vi "Initialize.vi"(8 "error in (no error)":errorcluster caption="错误输入（无错误）", 11 "VISA resource name in":refnum<visa-resource-name> caption="VISA资源名称输入") -> (0 "error out":errorcluster caption="错误输出", 3 "VISA resource name out":refnum<visa-resource-name> caption="VISA资源名称输出")   [LabVIEW 2015]
uses:
  <vilib>/Instr/_visa.llb/VISA Configure Serial Port (Instr).vi
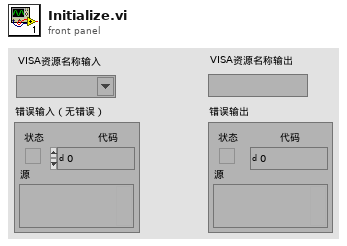
[diagram p1: front panel]
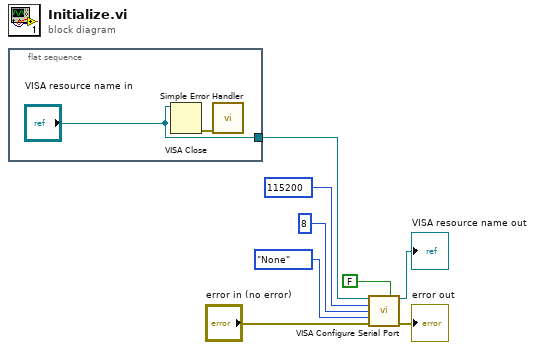
[diagram p0: block diagram]
diagram:
  n1 = flat-sequence {
    tunnel: ["VISA resource name in"] -> w4
    frame #0 {
      n2 = VISA Close(VISA resource name="VISA resource name in") -> (error out=w10:errorcluster)  [unwired: 1 in]
      n3 = call <vilib>:"Simple Error Handler.vi"("error in (no error)"=w10) -> ()  [unwired: 4 in, 5 out]
    }
  }
  n4 = call-poly "VISA Configure Serial Port"("VISA resource name"=w4, "Enable Termination\nChar (T)"=FALSE ("Enable Termination\nChar (T)"), "baud rate (9600)"=u32 115200, "data bits (8)"=u16 8, "parity (0:none)"=enum16{"None", "Odd", "Even", "Mark", "Space"}."None", "error in (no error)"="error in (no error)") -> ("VISA resource name out"=→"VISA resource name out":refnum<visa-resource-name>, "error out"=→"error out":errorcluster)  [unwired: 8 in]
